vi "GET_volumes_by_publisher.vi"(8 "error in (no error)":errorcluster) -> (0 "error out":errorcluster)   [LabVIEW 2024]
uses:
  <vilib>/addons/_JKI.lib/REST Client/classes/REST Client/HTTP Header.ctl
  <vilib>/NI/Advanced HTTP Client/Header--Combo Box.ctl
  <vilib>/addons/_JKI.lib/REST Client/classes/REST Client/REST Client.lvclass
  <vilib>/NI/Advanced HTTP Client/Session.lvclass
  <userlib>/_OpenG.lib/string/string.llb/openg_string.lvlib
panel:
  out "Response body":string
  in  "input 2":string
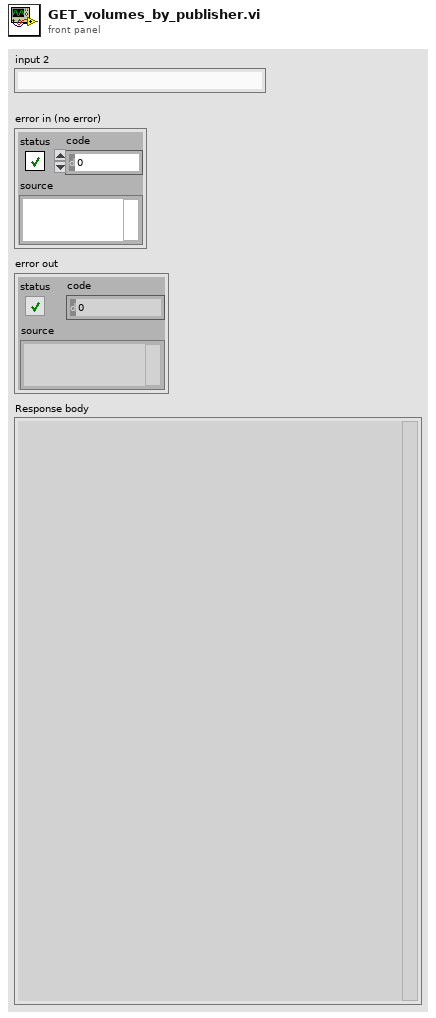
[diagram p1: front panel]
types:
  T1 = typedef "REST Client.lvlib/REST Client.lvclass/HTTP Header.ctl" = cluster{"header":T2, "value":string}
  T2 = typedef "lib_NI_Advanced HTTP Client.lvlib/Session.lvclass/Header--Combo Box.ctl" = string
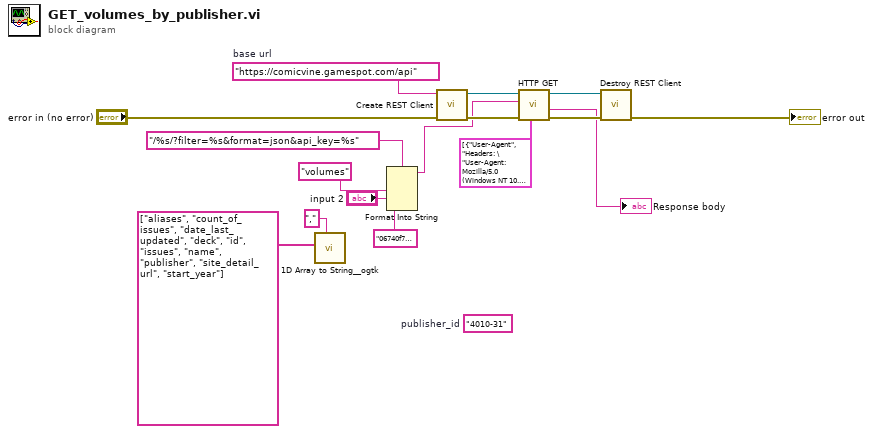
[diagram p0: block diagram]
diagram:
  (unwired) "4010-31"  # publisher_id
  w16 = "https://comicvine.gamespot.com/api"  # base url
  n1 = call <userlib>:"1D Array to String__ogtk.vi"("delimiter (Tab)"=",", "Array of Strings"=string[] ["aliases", "count_of_issues", "date_last_updated", "deck", "id", "issues", "name", "publisher", "site_detail_url", "start_year"]) -> ()  [unwired: 9 in, 1 out]
  n2 = Format Into String(format string="/%s/?filter=%s&format=json&api_key=%s", "volumes" ("resource"), "input 2", "06740f73403e0b211d597c50ea94c7f16ea5e8ea") -> (resulting string=w7:string)  [unwired: 2 in, 1 out]
  n3 = call <vilib>:"Create REST Client.vi"("error in (no error)"="error in (no error)", "Base URL"=w16) -> ("error out"=w13:errorcluster, "REST Client out"=w15:refnum<class "REST Client.lvclass">)  [unwired: 8 in]
  n4 = call-dynamic "HTTP GET.vi"("request specific headers"=T1[] [{"header"="User-Agent", "value"="Headers: \"User-Agent: Mozilla/5.0 (Windows NT 10.0; Win64; x64) AppleWebKit/537.36 (KHTML, like Gecko) Chrome/91.0.4472.101 Safari/537.36\""}], "error in (no error)"=w13, "Path"=w7, "REST Client in"=w15) -> ("error out"=w12:errorcluster, "Response body"=→"Response body":string, "REST Client out"=w14:refnum<class "REST Client.lvclass">)  [unwired: 2 in, 3 out]
  n5 = call-dynamic "Destroy REST Client.vi"("error in (no error)"=w12, "REST Client in"=w14) -> ("error out"=→"error out":errorcluster)  [unwired: 9 in]
